vi "rpc_tsmaster_call_system_api.vi"(8 "error in (no error)":errorcluster caption="错误输入（无错误）", 9 "AHandle":u32, 10 "API_param":T1, 11 "路径输入":path) -> (0 "error out":errorcluster caption="错误输出", 2 "function return":i32, 3 "路径输出":path)   [LabVIEW 2014]
doc: "After calling the location to create TSMaster Rpc client\nInput parameter AHHandle: TSMaster Rpc client handle\nAAPIName: System function name, \"app. creat_Systemnvar\" AArgCount: Number of function parameters\nAArgCapacity: Parameter string length\nAArgs: Parameter string array\nReturn value==0: Function execution successful\nOther values: Function execution failed"
uses:
  Typedef/RPC_API_param.ctl
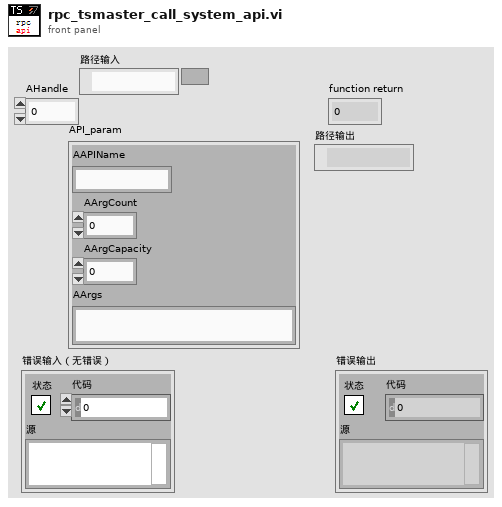
[diagram p1: front panel]
types:
  T1 = typedef "RPC_API_param.ctl" = cluster{"AAPIName":string, "AArgCount":i32, "AArgCapacity":i32, "AArgs":string}
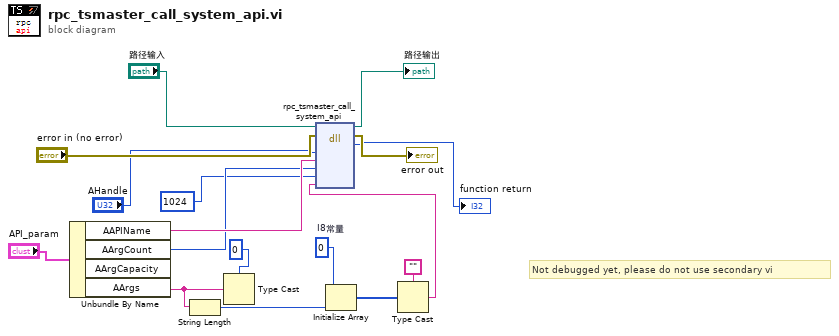
[diagram p0: block diagram]
diagram:
  w1 = i8 0  # I8常量
  # "Not debugged yet, please do not use secondary vi"
  n1 = Unbundle By Name("API_param") -> ("AAPIName"=w10:string, "AArgCount"=w9:i32, "AArgs"=w3:string)  [unwired: 1 out]
  n2 = String Length(string=w3) -> (length=w6:i32)
  n3 = Type Cast(type=u64 0 ("AArgs"), x=w3) -> ()  [unwired: 1 out]
  n4 = Initialize Array(w1, w6) -> (w5:i8[])
  n5 = Type Cast(type="" ("Empty String Constant"), x=w5) -> (*(type *) &x=w2:string)
  n6 = dll-call lib="D:/Program Files (x86)/TOSUN/TSMaster/bin/TSMaster.dll" fn="rpc_tsmaster_call_system_api"(path in="路径输入", error in="error in (no error)", "AHandle"="AHandle", "AAPIName"=w10, "AArgCount"=w9, "AArgCapacity"=1024, "AArgs"=w2) -> (path out=→"路径输出":path, error out=→"error out":errorcluster, "返回类型"=→"function return":i32)  [unwired: 6 in]
